vi "Active Option Update.vi"(8 "error in (no error)":errorcluster, 10 "Active Option":string, 11 "Normal Car Position Simulation View in":refnum<class "Normal Car Position Simulation View.lvclass">) -> (0 "error out":errorcluster, 3 "Normal Car Position Simulation View out":refnum<class "Normal Car Position Simulation View.lvclass">)   [LabVIEW 2019, in "Normal Car Position Simulation View.lvclass"]
uses:
  <vilib>/gpm_packages/@cs/Car-wash/Source/Normal Car Position Simulation View/Normal Car Position Simulation View/Normal Car Position Simulation View.lvclass
  C:/Program Files/National Instruments/LabVIEW 2019/vi.lib/gpm_packages/@cs/Car-wash/Source/Car Position Simulation View Definition/Car Position Simulation View Definition/Car Position Simulation View Definition.lvclass
  <vilib>/gpm_packages/@cs/Car-wash/Source/Car Position Simulation View Definition/Car Position Simulation View Definition/Car Position Simulation View Definition.lvclass/Car Position Simulation View Definition.ctl
  <vilib>/gpm_packages/@cs/Car-wash/Source/Car Position Simulation View Definition/Car Position Simulation View Definition/Car Position Simulation View Definition.lvclass
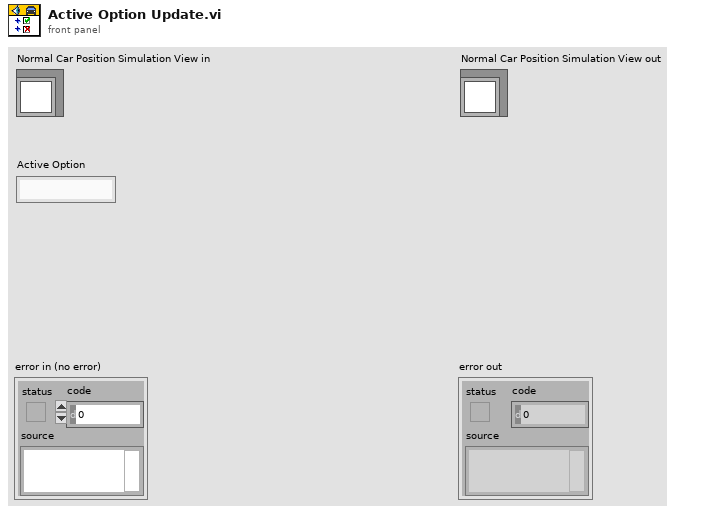
[diagram p1: front panel]
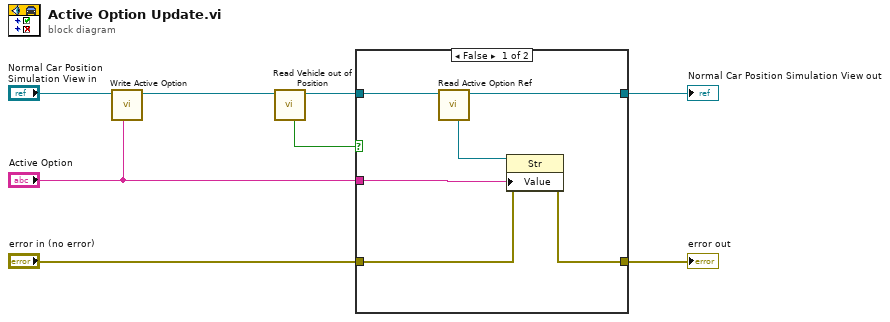
[diagram p0: block diagram]
diagram:
  n1 = call <vilib>:"Write Active Option.vi"("Active Option"="Active Option", "Car Position Simulation View Definition in"="Normal Car Position Simulation View in") -> ("Car Position Simulation View Definition out"=w3:refnum<class "Normal Car Position Simulation View.lvclass">)  [unwired: 9 in]
  n2 = call <vilib>:"Read Vehicle out of Position.vi"("Car Position Simulation View Definition in"=w3) -> ("Car Position Simulation View Definition out"=w2:refnum<class "Normal Car Position Simulation View.lvclass">, "Vehicle out of Position"=w1:bool)  [unwired: 9 in]
  n3 = case shown="False" w1 {
    tunnel: [w14 w16] -> w8
    tunnel: "error in (no error)" -> [w12 w15]
    tunnel: [w11 w15] -> w6
    tunnel: "Active Option" -> [w10 _]
    tunnel: w2 -> [w9 w16]
    frame False {
      n4 = call <vilib>:"Read Active Option Ref.vi"("Car Position Simulation View Definition in"=w9) -> ("Car Position Simulation View Definition out"=w14:refnum<class "Normal Car Position Simulation View.lvclass">, "Active Option Ref"=w13:refnum<vi>)  [unwired: 9 in]
      n5 = property class="Str"(reference=w13, error in=w12, "Value"=w10) -> (error out=w11:errorcluster)  [unwired: 1 out]
    }
    frame True {
    }
  }
  "error out" <- w6
  "Normal Car Position Simulation View out" <- w8
